vi "Insert_all_volumes_from_json.vi"() -> ()   [LabVIEW 2024]
uses:
  <vilib>/drjdpowell/SQLite Library/SQL Connection/Open (path).vi
  <vilib>/drjdpowell/SQLite Library/SQL Connection/Open (string).vi
  <vilib>/AdvancedString/Path To Command Line String.vi
  <vilib>/drjdpowell/SQLite Library/SQL Connection/Execute SQL (No results).vi
  <vilib>/drjdpowell/SQLite Library/SQL Connection/Connection.lvclass
  <vilib>/drjdpowell/SQLite Library/SQLite.lvlib
  <userlib>/_OpenG.lib/string/string.llb/openg_string.lvlib
  <vilib>/addons/_JKI.lib/REST Client/classes/REST Client/REST Client.lvclass
panel:
  out "progress":i32(slide) scale=0.0..2851.0
  in  "volume_path":path=path "D:/Comics/data/cv_volumes"
  out "error out":errorcluster
  in  "db path":path=path "D:/Comics/data/comicvine.db"
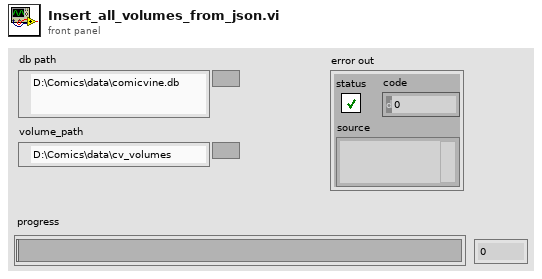
[diagram p1: front panel]
types:
  T1 = typedef "local_volume.ctl" = cluster{"id":i32, "name":string, "sortable_name":string, "aliases":string[], "description":string, "site_detail_url":string, "count_of_issues":i32, "start_year":i32, "publisher_id":i32, "issue_ids":i32[], "date_last_updated":timestamp, "volume":i32, "cv_id":string}
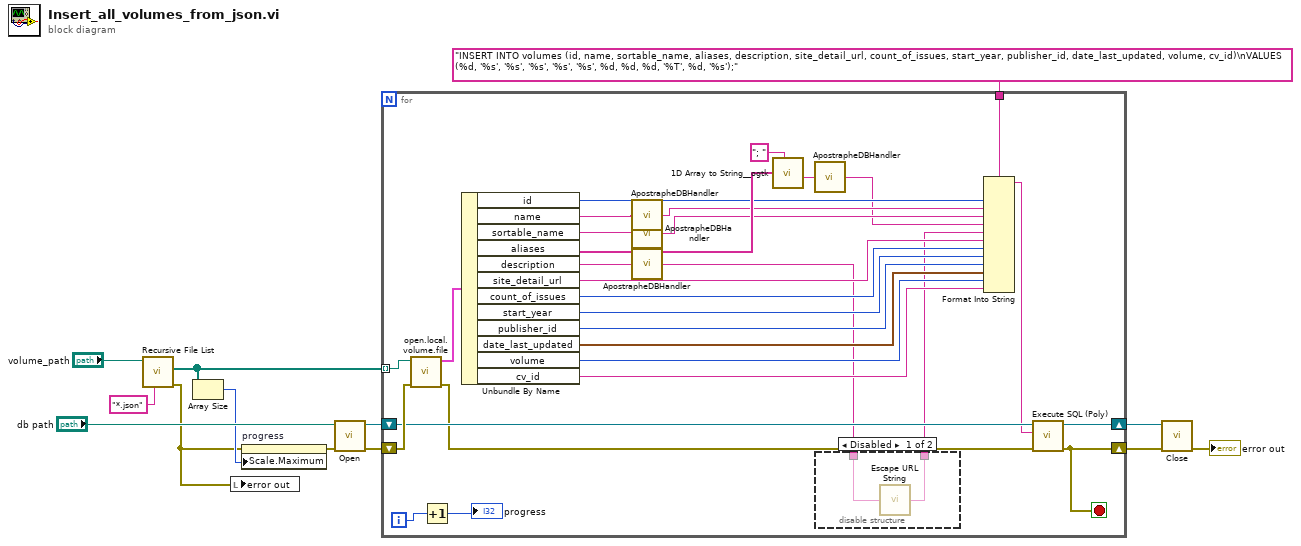
[diagram p0: block diagram]
diagram:
  n1 = call <vilib>:"Recursive File List.vi"("pattern"="*.json", "Folder Path"="volume_path") -> ("error out"=w1:errorcluster, "All Files in Dir"=w6:path[])  [unwired: 5 in, 3 out]
  n2 = Array Size(array=w6) -> (size(s)=w4:i32)
  n3 = local write "error out"(w1) -> ()
  n4 = property on="progress" class="Slide (strict)"(error in=w1, "Scale.Maximum"=w4) -> (error out=w5:errorcluster)  [unwired: 1 in, 1 out]
  n5 = call-poly <vilib>:"Open.vi"("error in (no error)"=w5, "db file"="db path") -> ("error out"=w8:errorcluster, "SQLite Connection"=w7:refnum<class "Connection.lvclass">)  [unwired: 8 in]
  n6 = for {
    tunnel: w6 -> [w42] mode=indexing
    tunnel: "INSERT INTO volumes (id, name, sortable_name, aliases, description, site_detail_url, count_of_issues, start_year, publisher_id, date_last_updated, volume, cv_id)\nVALUES (%d, '%s', '%s', '%s', '%s', '%s', %d, %d, %d, '%T', %d, '%s');" -> [w38]
    shift-right: [w23] -> w2
    shift-left: w8 -> [w43]
    shift-right: [w27] -> w3
    shift-left: w7 -> [w29]
    i -> [w25]
    stop <- w23 stop-if-true
    n7 = call "open.local.volume.file.vi"("error in (no error)"=w43, "volume json"=w42) -> ("error out"=w28:errorcluster, "volume"=w41:T1)  [unwired: 8 in]
    n8 = Increment(x=w25) -> (x+1=→"progress":i32)
    n9 = Unbundle By Name(w41) -> ("id"=w37:i32, "name"=w21:string, "sortable_name"=w19:string, "aliases"=w40:string[], "description"=w15:string, "site_detail_url"=w36:string, "count_of_issues"=w35:i32, "start_year"=w34:i32, "publisher_id"=w33:i32, "date_last_updated"=w32:timestamp, "volume"=w31:i32, "cv_id"=w30:string)
    n10 = call "ApostrapheDBHandler.vi"("string in"=w21) -> ("string out"=w20:string)
    n11 = call "ApostrapheDBHandler.vi"("string in"=w19) -> ("string out"=w18:string)
    n12 = call "ApostrapheDBHandler.vi"("string in"=w15) -> ("string out"=w14:string)
    n13 = call <userlib>:"1D Array to String__ogtk.vi"("delimiter (Tab)"="; ", "Array of Strings"=w40) -> ("delimited string"=w16:string)  [unwired: 9 in]
    n14 = call "ApostrapheDBHandler.vi"("string in"=w16) -> ("string out"=w17:string)
    n15 = disable-structure shown="Disabled" {
      disable-tunnel: w14 -> [w45 w46]
      disable-tunnel: [w44 w46] -> w22
      frame Disabled {
        n16 = call <vilib>:"Escape URL String.vi"("Unescaped URL string in"=w45) -> ("Escaped URL string out"=w44:string)
      }
      frame Enabled {
      }
    }
    n17 = Format Into String(format string=w38, w37, w20, w18, w17, w22, w36, w35, w34, w33, w32, w31, w30) -> (resulting string=w26:string)  [unwired: 2 in, 1 out]
    n18 = call-poly <vilib>:"Execute SQL (Poly).vi"("error in (no error)"=w28, "SQL"=w26, "SQLite Connection in"=w29) -> ("error out"=w23:errorcluster, "SQLite Connection"=w27:refnum<class "Connection.lvclass">)  [unwired: 7 in]
  }
  n19 = call-dynamic "Close.vi"("error in (no error)"=w2, "SQLite Connection in"=w3) -> ("error out"=→"error out":errorcluster)  [unwired: 9 in]
